vi "Move Z.vi"(8 "Device and Axis":string[][](array[string]), 9 "Linear Microstep Size":dbl, 10 "Z (mm)":dbl, 11 "VISA resource name":refnum<visa-resource-name>) -> (3 "VISA resource name out":refnum<visa-resource-name>)   [LabVIEW 2018, in "Stage Actor.lvlib"]
uses:
  Stage Actor.lvlib
  <instrlib>/Zaber A Series/Zaber A Series.lvlib
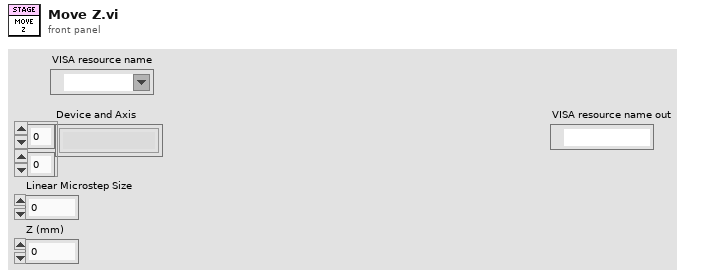
[diagram p1: front panel]
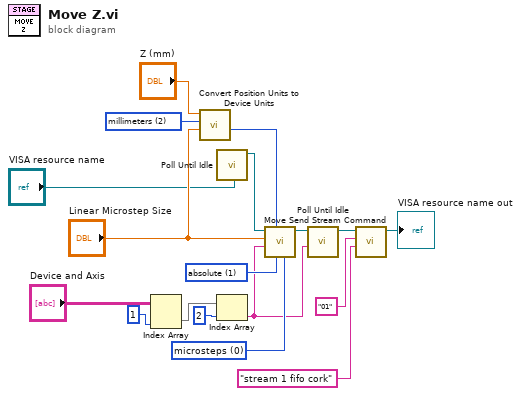
[diagram p0: block diagram]
diagram:
  w8 = u16 0 items=["microsteps", "microns", "millimeters", "inches", "degrees"] ("Units (0: microsteps)")
  w9 = u16 1 items=["relative", "absolute"] ("Movement Type (0: relative)")
  w13 = u16 2 items=["microsteps", "microns", "millimeters", "inches", "degrees"] ("Units (0: microsteps)")
  n1 = Index Array(array="Device and Axis", index (col)=1 ("disabled index (col)")) -> (element=w11:string[])  [unwired: 1 in]
  n2 = call <instrlib>:"Convert Position Units to Device Units.vi"("Microstep Size (0)"="Linear Microstep Size", "Units (0: microsteps)"=w13, "Position (0)"="Z (mm)") -> ("Device Position (64-bit)"=w1:i64)  [unwired: 6 in, 2 out]
  n3 = call <instrlib>:"Poll Until Idle.vi"("VISA resource name"="VISA resource name") -> ("VISA resource name out"=w5:refnum<visa-resource-name>)  [unwired: 9 in, 1 out]
  n4 = Index Array(array=w11, index=2) -> (element=w6:string)
  n5 = call <instrlib>:"Move.vi"("Units (0: microsteps)"=w8, "Movement Type (0: relative)"=w9, "Move Distance (0)"=w1, "Device and Axis"=w6, "Microstep Size (0)"="Linear Microstep Size", "VISA resource name"=w5) -> ("VISA resource name out"=w7:refnum<visa-resource-name>)  [unwired: 4 in, 1 out]
  n6 = call <instrlib>:"Poll Until Idle.vi"("Device and Axis"=w6, "VISA resource name"=w7) -> ("VISA resource name out"=w3:refnum<visa-resource-name>)  [unwired: 8 in, 1 out]
  n7 = call <instrlib>:"Send Stream Command.vi"("Command"="stream 1 fifo cork", "Device Number"="01", "VISA resource name"=w3) -> ("VISA resource name out"=→"VISA resource name out":refnum<visa-resource-name>)  [unwired: 7 in, 1 out]
